vi "BRig_Host__Loop_Producer__UploadClosedLoop__v5.vi"(1 "input_arrayBuffer_length":i32, 2 "input_arrayBuffer":u16[][](array[numeric]), 4 "input_cmdList":bool, 5 "input_cmdList":u16[][](array[numeric]), 6 "input_webdav_status":bool, 8 "session handle":T1, 9 "testNewLaserSettings":bool, 11 "input_array_LaserSettings":u16[](array[numeric])) -> (12 "Sent":bool, 15 "output_arrayBuffer_length":i32, 16 "output_arrayBuffer":u16[][](array[numeric]))   [LabVIEW 2014]
uses:
  <vilib>/WebDAVClient/Advanced/SessionHandle.ctl
  <vilib>/Utility/file.llb/Write To Spreadsheet File (I64).vi
  <vilib>/WebDAVClient/Advanced/Put File.vi
  <vilib>/WebDAVClient/NI_WebDAV.lvlib
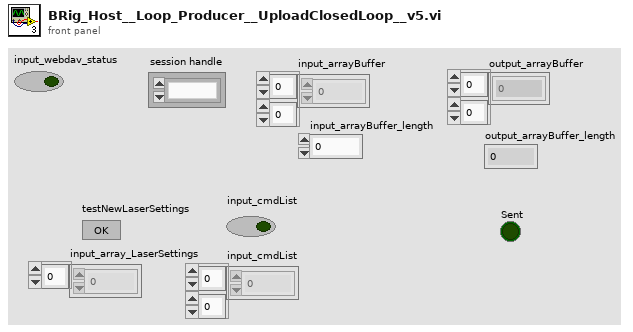
[diagram p1: front panel]
types:
  T1 = typedef "NI_WebDAV.lvlib/SessionHandle.ctl" = refnum<k1>
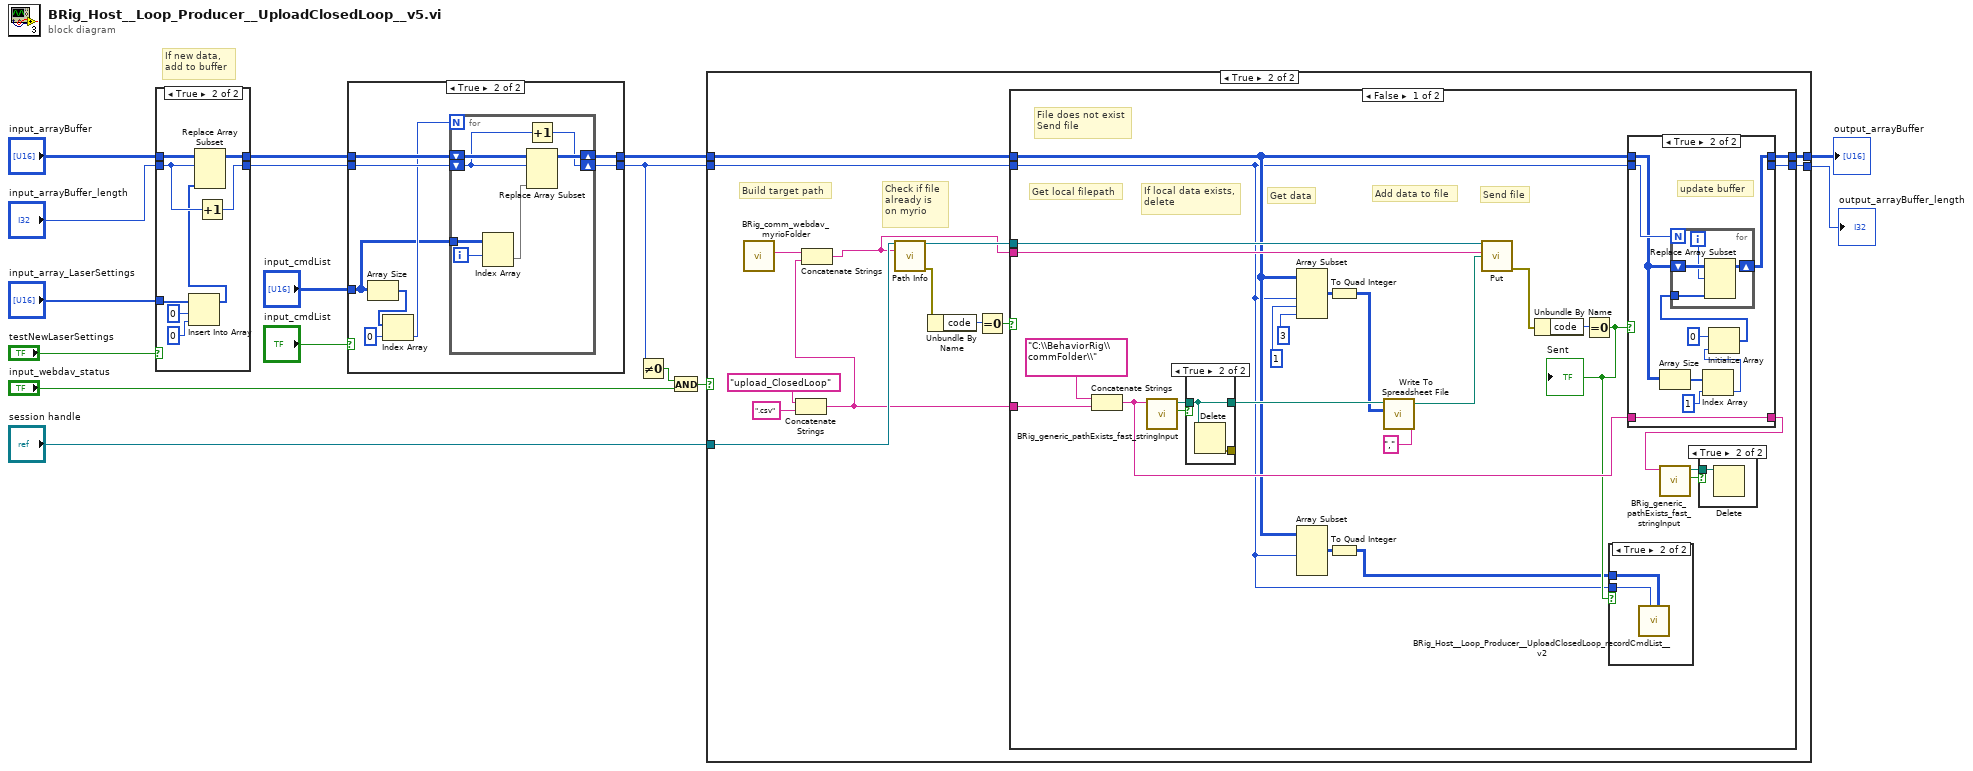
[diagram p0: block diagram]
diagram:
  # "If new data,\nadd to buffer"
  n1 = case shown="True" "testNewLaserSettings" {
    tunnel: "input_arrayBuffer" -> [w18 w26]
    tunnel: [w18 w25] -> w6
    tunnel: [w17 w23] -> w4
    tunnel: "input_arrayBuffer_length" -> [w17 w24]
    tunnel: "input_array_LaserSettings" -> [_ w22]
    frame False {
    }
    frame True {
      n2 = Insert Into Array(array=w22, index=0, new element=u16 0 ("new element/subarray")) -> (w19:u16[])
      n3 = Replace Array Subset(array=w26, new element=w19, index (row)=w24) -> (w25:u16[][])  [unwired: 1 in]
      n4 = Increment(x=w24) -> (x+1=w23:i32)
    }
  }
  n5 = case shown="True" "input_cmdList" {
    tunnel: w6 -> [w28 w34]
    tunnel: [w28 w33] -> w5
    tunnel: w4 -> [w27 w32]
    tunnel: [w27 w31] -> w3
    tunnel: "input_cmdList" -> [_ w29]
    frame False {
    }
    frame True {
      n6 = Array Size(array=w29) -> (size(s)=w36:i32[])
      n7 = Index Array(array=w36, index=0) -> (element=w30:i32)
      n8 = for {
        N: w30 -> [_]
        shift-right: [w40] -> w33
        shift-left: w34 -> [w41]
        shift-right: [w39] -> w31
        shift-left: w32 -> [w38]
        tunnel: w29 -> [w43]
        i -> [w42]
        n9 = Index Array(array=w43, index (row)=w42) -> (element=w37:u16[])  [unwired: 1 in]
        n10 = Increment(x=w38) -> (x+1=w39:i32)
        n11 = Replace Array Subset(array=w41, new element=w37, index (row)=w38) -> (w40:u16[][])  [unwired: 1 in]
      }
    }
  }
  n12 = Not Equal To 0?(x=w3) -> (x != 0?=w8:bool)
  n13 = And(x=w8, y="input_webdav_status") -> (x .and. y?=w7:bool)
  n14 = case shown="True" w7 {
    tunnel: "session handle" -> [_ w54]
    tunnel: w5 -> [w45 w52]
    tunnel: [w45 w51] -> w15
    tunnel: w3 -> [w44 w50]
    tunnel: [w44 w49] -> w14
    frame False {
    }
    frame True {
      # "Check if file\nalready is\non myrio"
      # "Build target path"
      n15 = call "BRig_comm_webdav_myrioFolder.vi"() -> ("output_myrioFolder"=w57:string)  [unwired: 11 in]
      n16 = Concatenate Strings("upload_ClosedLoop" ("string"), ".csv" ("string")) -> (w48:string)
      n17 = Concatenate Strings(w57, w48) -> (w46:string)
      n18 = call <vilib>:"Path Info.vi"("session handle"=w54, "relative uri"=w46) -> ("session handle out"=w47:T1, "error out"=w55:errorcluster)  [unwired: 10 in, 2 out]
      n19 = Unbundle By Name(w55) -> ("code"=w56:i32)
      n20 = Equal To 0?(x=w56) -> (x = 0?=w53:bool)
      n21 = case shown="False" w53 {
        tunnel: w52 -> [w64 w109]
        tunnel: [w77 w109] -> w51
        tunnel: w50 -> [w62 w108]
        tunnel: [w76 w108] -> w49
        tunnel: w48 -> [w85 _]
        tunnel: w47 -> [w79 _]
        tunnel: w46 -> [w78 _]
        frame False {
          # "Send file"
          # "Add data to file"
          # "Get data"
          # "If local data exists,\ndelete"
          # "Get local filepath"
          # "File does not exist\nSend file"
          n22 = Concatenate Strings("C:\\BehaviorRig\\commFolder\\", w85) -> (w72:string)
          n23 = call "BRig_generic_pathExists_fast_stringInput.vi"("input_filePath"=w72) -> ("output_Iexist"=w84:bool, "output_filePath"=w83:path)  [unwired: 8 in, 1 out]
          n24 = case shown="True" w84 {
            tunnel: w83 -> [w105 w106]
            tunnel: [_ w107] -> _
            tunnel: [w105 w106] -> w82
            frame False {
            }
            frame True {
              n25 = Delete(path (use dialog)=w106) -> (error out=w107:errorcluster)  [unwired: 4 in, 2 out]
            }
          }
          n26 = Array Subset(array=w64, length (row)=w62, index (col)=1 ("index"), length (col)=3 ("length")) -> (w69:u16[][])  [unwired: 1 in]
          n27 = Array Subset(array=w64, length (row)=w62) -> (w65:u16[][])  [unwired: 3 in]
          n28 = To Quad Integer(1:w69) -> (0:w66:i64[][])
          n29 = To Quad Integer(1:w65) -> (0:w63:i64[][])
          n30 = call-poly <vilib>:"Write To Spreadsheet File.vi"("delimiter (\\t)"="," ("delimiter (\\t)"), "2D data"=w66, "file path (dialog if empty)"=w82) -> ("new file path (Not A Path if cancelled)"=w75:path)  [unwired: 5 in]
          n31 = call-poly <vilib>:"Put.vi"("session handle"=w79, "relative uri"=w78, "local file path"=w75) -> ("error out"=w81:errorcluster)  [unwired: 10 in, 2 out]
          n32 = Unbundle By Name(w81) -> ("code"=w80:i32)
          n33 = Equal To 0?(x=w80) -> (x = 0?=w67:bool)
          "Sent" <- w67
          n34 = case shown="True" w67 {
            tunnel: w62 -> [_ w87]
            tunnel: w63 -> [_ w86]
            frame False {
            }
            frame True {
              n35 = call "BRig_Host__Loop_Producer__UploadClosedLoop_recordCmdList__v2.vi"("input_newData"=w86, "input_n"=w87) -> ()  [unwired: 10 in]
            }
          }
          n36 = case shown="True" w67 {
            tunnel: w64 -> [w91 w95]
            tunnel: [w91 w93] -> w77
            tunnel: w62 -> [w90 w100]
            tunnel: [w90 _] -> w76
            tunnel: w72 -> [w89 w92]
            tunnel: [w89 w92] -> w71
            frame False {
            }
            frame True {
              # "update buffer"
              n37 = Array Size(array=w95) -> (size(s)=w99:i32[])
              n38 = Index Array(array=w99, index=1) -> (element=w97:i32)
              n39 = Initialize Array(u16 0 ("element"), w97) -> (w94:u16[])
              n40 = for {
                N: w100 -> [_]
                shift-right: [w103] -> w93
                shift-left: w95 -> [w104]
                tunnel: w94 -> [w101]
                i -> [w102]
                n41 = Replace Array Subset(array=w104, new element=w101, index (row)=w102) -> (w103:u16[][])  [unwired: 1 in]
              }
            }
          }
          n42 = call "BRig_generic_pathExists_fast_stringInput.vi"("input_filePath"=w71) -> ("output_Iexist"=w73:bool, "output_filePath"=w74:path)  [unwired: 8 in, 1 out]
          n43 = case shown="True" w73 {
            tunnel: w74 -> [_ w88]
            frame False {
            }
            frame True {
              n44 = Delete(path (use dialog)=w88) -> ()  [unwired: 4 in, 3 out]
            }
          }
        }
        frame True {
          # "File does exist\nWait for myrio to process it"
        }
      }
    }
  }
  "output_arrayBuffer" <- w15
  "output_arrayBuffer_length" <- w14
